vi "niFpgaMemoryEmulationDramWriteAndRequestDataRefIn.vi"(0 "address":u32, 1 "Name":variant, 5 "data":i32, 7 "write":bool, 9 "input valid":bool, 11 "error in (no error)":errorcluster, 12 "byte enables":i64, 13 "Node Link":cluster{"VIRef":refnum<vi>, "UID":i32}) -> (10 "ready for input":bool, 15 "error out":errorcluster)   [LabVIEW 2017]
uses:
  <vilib>/rvi/DataTransferAndStorage/Container/Common/niFpgaContainerMetaDataKey.ctl
  <instcachedir>/0/niFpgaMemoryFastEmulationDramWriteAndRequestData_E252DB80A3454BECA2A169E9D5D57AEC.lvgen/niFpgaMemoryFastEmulationDramWriteAndRequestData_E252DB80A3454BECA2A169E9D5D57AEC_000.vi
  <instcachedir>/0/niFpgaMemoryEmulationDramWriteAndRequestData_CD4074A3DA3C46109C257B40B1EDF874.lvgen/niFpgaMemoryEmulationDramWriteAndRequestData_CD4074A3DA3C46109C257B40B1EDF874_000.vi
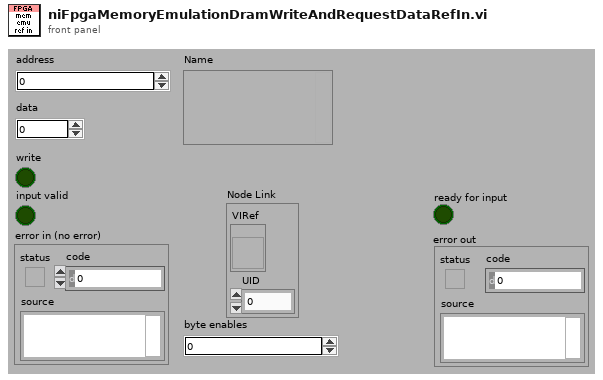
[diagram p1: front panel]
types:
  T1 = typedef "niFpgaContainerMetaDataKey.ctl" = enum16{"FPGA FIFO", "FPGA Memory", "FPGA Register", "FPGA Handshake"}
  T2 = typedef "niFpgaContainerState.ctl" = cluster{"displayName":string, "hardwareName":string, "dataType":T3, "elementTypeDescriptor":variant, "terminalTypeDescriptor":variant, "requestedNumberOfElements":u32, "memoryType":T4, "arbitrationForInterfaceA":T5, "numberOfElementsPerRead":u32, "arbitrationForInterfaceB":T5, "numberOfElementsPerWrite":u32, "VI_Defined":bool, "type":T6, "initializationParameters":T7, "disableOnOverflow/Underflow":bool, "interfaceConfiguration":T8, "controlLogic":T9, "actualNumberOfElements":u32, "dramSelection":string, "dramMaxOustandingRequests":i32, "dramIncludeByteEnables":bool, "dramGrantTime":u32, "fullEmulation":bool, "memoryInMultipleClockDomains":bool, "memoryLatency":T10}
  T3 = typedef "niFpgaDataTypeControl.ctl" = enum32{"Boolean", "I8", "I16", "I32", "I64", "U8", "U16", "U32", "U64", "FXP", "CustomControl", "SGL"}
  T4 = typedef "niFpgaContainerImplementationControl.ctl" = enum16{"Flip-Flops", "Look-Up Table", "Block Memory", "DRAM"}
  T5 = typedef "niFpgaContainerArbitrationOptionsControl.ctl" = enum16{"Always Arbitrate", "Arbitrate if Multiple Requestors Only", "Never Arbitrate"}
  T6 = typedef "niFpgaTransferTypeControl.ctl" = enum16{"Target-Scoped", "Host to Target - DMA", "Target to Host - DMA", "Peer to Peer Reader", "Peer to Peer Writer", "Bidirectional"}
  T7 = typedef "niFpgaContainerInitializationParameters.ctl" = cluster{"initialized":bool, "VI_Path":path, "initialData":variant}
  T8 = typedef "niFpgaMemoryInterfaceConfiguration.ctl" = enum16{"Read A-Write B", "Read A-Read B"}
  T9 = typedef "niFpgaFifoControlLogicControl.ctl" = enum16{"Slice Fabric", "Target Optimal", "Built-in"}
  T10 = typedef "niFpgaContainerMemoryLatencyControl.ctl" = u16
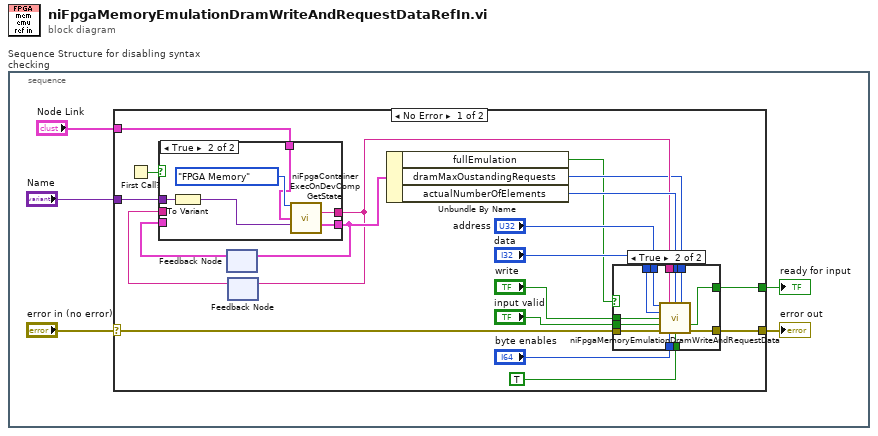
[diagram p0: block diagram]
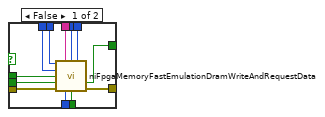
[diagram p2: hidden frame]
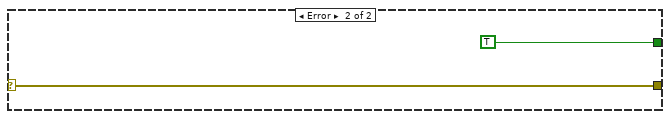
[diagram p4: hidden frame]
diagram:
  n1 = stacked-sequence "Sequence Structure for disabling syntax checking" {
    frame #0 {
      n2 = case shown="No Error" "error in (no error)" {
        selector: "error in (no error)" -> [w12 w58]
        tunnel: [w22 w58] -> w2
        tunnel: "Name" -> [w18 _]
        tunnel: [w8 TRUE ("ready for input")] -> w5
        tunnel: "Node Link" -> [w6 _]
        frame No Error {
          n3 = First Call?() -> (First Call?: T/F=w20:bool)
          n4 = feedback #1() -> (w15:T2)  [unwired: 1 out]
          n5 = feedback #2() -> (w13:string)  [unwired: 1 out]
          n6 = case shown="True" w20 {
            tunnel: w18 -> [_ w56]
            tunnel: [w50 w52] -> w16
            tunnel: w15 -> [w50 _]
            tunnel: [w49 w53] -> w14
            tunnel: w13 -> [w49 _]
            tunnel: w6 -> [_ w51]
            frame False {
            }
            frame True {
              n7 = To Variant(anything=w56) -> (Variant=w55:variant)
              n8 = call <vilib>:"niFpgaContainerExecOnDevCompGetState.vi"("containerMetaDataKey"=niFpgaContainerMetaDataKey."FPGA Memory", "Node Link"=w51, "name"=w55) -> ("Unique  Name"=w53:string, "containerState"=w52:T2)  [unwired: 3 in, 8 out]
            }
          }
          n9 = feedback-in #1(w16) -> ()
          n10 = feedback-in #2(w14) -> ()
          n11 = Unbundle By Name(w16) -> ("fullEmulation"=w7:bool, "dramMaxOustandingRequests"=w10:i32, "actualNumberOfElements"=w19:u32)
          n12 = case shown="True" w7 {
            tunnel: "address" -> [w36 w48]
            tunnel: "write" -> [w35 w47]
            tunnel: [w34 w46] -> w22
            tunnel: "data" -> [w33 w45]
            tunnel: w19 -> [w32 w44]
            tunnel: TRUE ("ref in wired") -> [w31 w43]
            tunnel: w14 -> [w30 w42]
            tunnel: w12 -> [w29 w41]
            tunnel: "byte enables" -> [w28 w40]
            tunnel: w10 -> [w27 w39]
            tunnel: "input valid" -> [w26 w38]
            tunnel: [w25 w37] -> w8
            frame False {
              n13 = call-generic <vilib>:"niFpgaMemoryFastEmulationDramWriteAndRequestData.vi"("address"=w36, "name"=w30, "number of elements"=w32, "fifo size"=w27, "data"=w33, "write"=w35, "input valid"=w26, "error in (no error)"=w29, "byte enables"=w28, "ref in wired"=w31) -> ("ready for input"=w25:bool, "error out"=w34:errorcluster)  [unwired: 4 in]
            }
            frame True {
              n14 = call-generic <vilib>:"niFpgaMemoryEmulationDramWriteAndRequestData.vi"("address"=w48, "name"=w42, "number of elements"=w44, "fifo size"=w39, "data"=w45, "write"=w47, "input valid"=w38, "error in (no error)"=w41, "byte enables"=w40, "ref in wired"=w43) -> ("ready for input"=w37:bool, "error out"=w46:errorcluster)  [unwired: 4 in]
            }
          }
        }
        frame Error {
        }
      }
      "error out" <- w2
      "ready for input" <- w5
    }
  }
